vi "Read XML_Extra Checks_Check Parameter startBit Tx.vi"(8 "error in (no error)":errorcluster, 11 "Channels In":T1[](array[typedef])) -> (0 "error out":errorcluster)   [LabVIEW 2016]
doc: "This VI checks that for a given Hardware Channel, all parameters have a unique combination of Parameter settings: Hardware Channel, Label Decimal and Parameter Name. If there are multiple duplicates, the function returns all duplicates."
uses:
  XML_Channel.ctl
  XML_Label.ctl
  XML_Parameter.ctl
  <userlib>/_OpenG.lib/array/array.llb/Filter 1D Array with Scalar (Boolean)__ogtk.vi
panel:
  out "Error Source":string
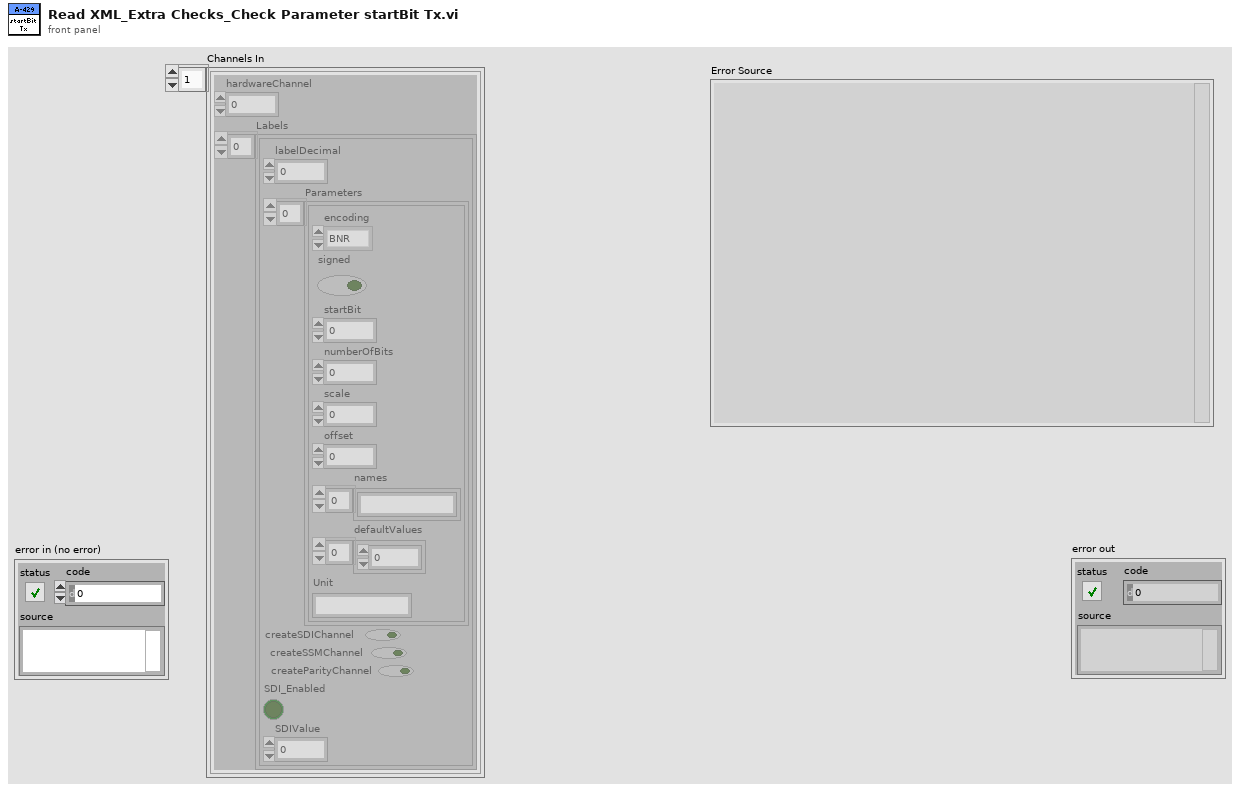
[diagram p1: front panel]
types:
  T1 = typedef "XML_Channel.ctl" = cluster{"hardwareChannel":i32, "Labels":T2[]}
  T2 = typedef "XML_Label.ctl" = cluster{"labelDecimal":i32, "Parameters":T3[], "createSDIChannel":bool, "createSSMChannel":bool, "createParityChannel":bool, "SDI_Enabled":bool, "SDIValue":u8}
  T3 = typedef "XML_Parameter.ctl" = cluster{"encoding":enum16{"BNR", "BCD", "Discrete"}, "signed":bool, "startBit":i32, "numberOfBits":i32, "scale":dbl, "offset":dbl, "names":string[], "defaultValues":dbl[], "Unit":string}
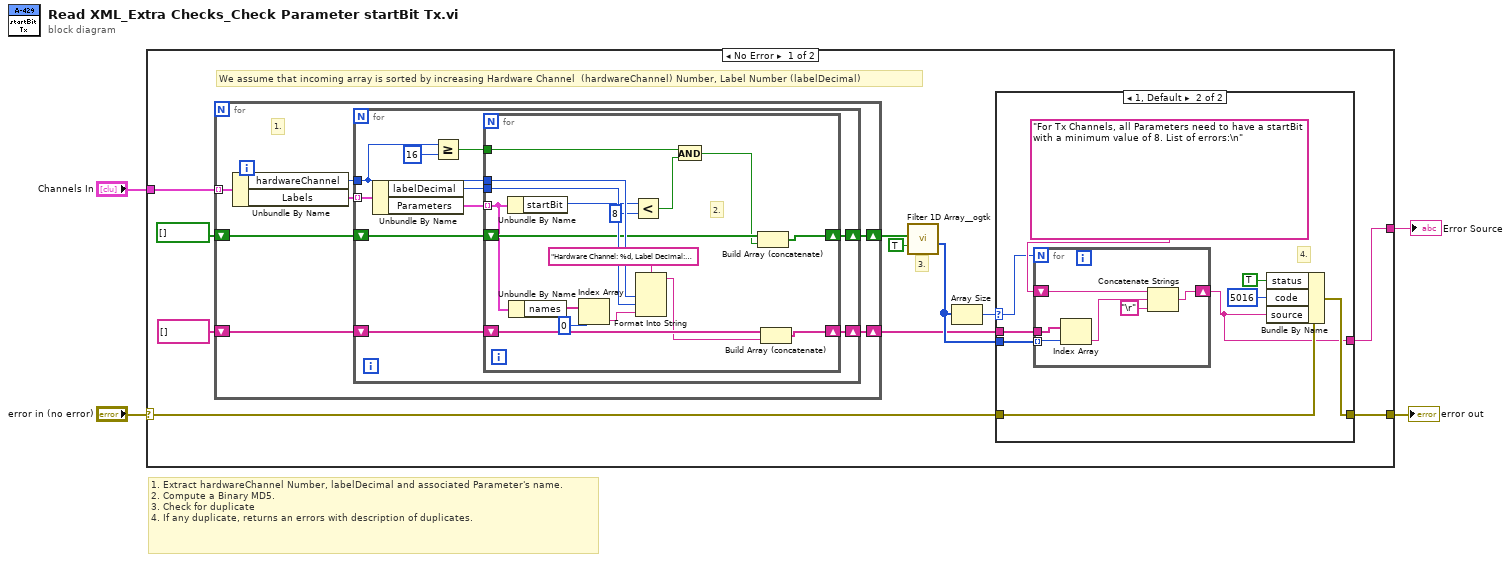
[diagram p0: block diagram]
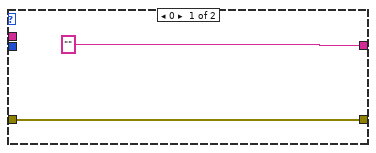
[diagram p2: hidden frame]
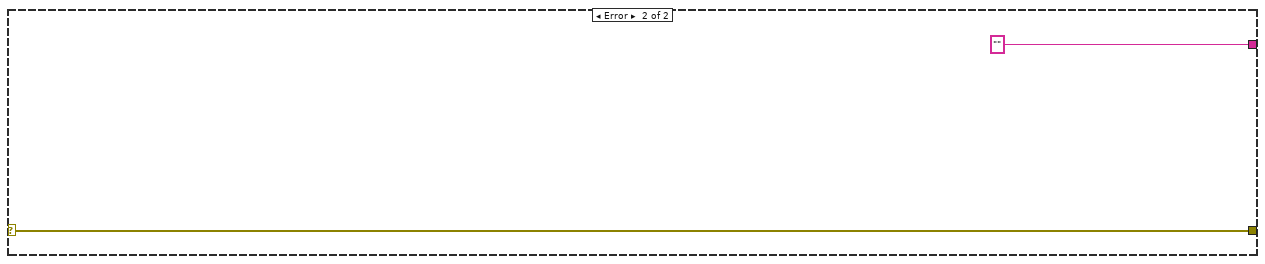
[diagram p3: hidden frame]
diagram:
  # "1. Extract hardwareChannel Number, labelDecimal and associated Parameter's name.\n2. Compute a Binary MD5.\n3. Check for duplicate\n4. If any duplicate, returns an errors with description of duplicates."
  n1 = case shown="No Error" "error in (no error)" {
    selector: "error in (no error)" -> [w14 w68]
    tunnel: [w11 w68] -> w3
    tunnel: "Channels In" -> [w13 _]
    tunnel: [w10 ""] -> w1
    frame No Error {
      # "3."
      # "We assume that incoming array is sorted by increasing Hardware Channel  (hardwareChannel) Number, Label Number (labelDecimal)"
      n2 = for {
        tunnel: w13 -> [w39] mode=indexing
        shift-right: [w35] -> w6
        shift-left: bool[] [] -> [w36]
        shift-right: [w33] -> w8
        shift-left: string[] [] -> [w34]
        # "1."
        n3 = Unbundle By Name(w39) -> ("hardwareChannel"=w38:i32, "Labels"=w37:T2[])
        n4 = for {
          tunnel: w38 -> [w42]
          tunnel: w37 -> [w49] mode=indexing
          shift-right: [w46] -> w35
          shift-left: w36 -> [w47]
          shift-right: [w43] -> w33
          shift-left: w34 -> [w44]
          n5 = Unbundle By Name(w49) -> ("labelDecimal"=w48:i32, "Parameters"=w45:T3[])
          n6 = Greater Or Equal?(x=w42, y=16) -> (x >= y?=w40:bool)
          n7 = for {
            tunnel: w42 -> [w66]
            tunnel: w48 -> [w65]
            shift-right: [w63] -> w46
            shift-left: w47 -> [w64]
            tunnel: w45 -> [w60] mode=indexing
            shift-right: [w61] -> w43
            shift-left: w44 -> [w62]
            tunnel: w40 -> [w54]
            # "2."
            n8 = Unbundle By Name(w60) -> ("startBit"=w53:i32)
            n9 = Unbundle By Name(w60) -> ("names"=w57:string[])
            n10 = Index Array(array=w57, index=0) -> (element=w56:string)
            n11 = Less?(x=w53, y=8) -> (x < y?=w51:bool)
            n12 = Format Into String(format string="Hardware Channel: %d, Label Decimal: %d, Name: %s", w66, w65, w56) -> (resulting string=w58:string)  [unwired: 2 in, 1 out]
            n13 = And(x=w54, y=w51) -> (x .and. y?=w50:bool)
            n14 = Build Array (concatenate)(w64, w50) -> (w63:bool[])
            n15 = Build Array (concatenate)(w62, w58) -> (w61:string[])
          }
        }
      }
      n16 = call-poly <userlib>:"Filter 1D Array__ogtk.vi"("items to filter"=TRUE, "array"=w6) -> ("filtered item indices"=w12:i32[])  [unwired: 4 in, 1 out]
      n17 = Array Size(array=w12) -> (size(s)=w15:i32)
      n18 = case shown="1, Default" w15 {
        selector: w15 -> [_ w21]
        tunnel: w14 -> [w17 w26]
        tunnel: w12 -> [_ w20]
        tunnel: [w17 w25] -> w11
        tunnel: ["" w19] -> w10
        tunnel: w8 -> [_ w18]
        frame 0 {
        }
        frame 1, Default {
          # "4."
          n19 = for {
            N: w21 -> [_]
            shift-right: [w31] -> w19
            shift-left: "For Tx Channels, all Parameters need to have a startBit with a minimum value of 8. List of errors:\n" -> [w32]
            tunnel: w20 -> [w30] mode=indexing
            tunnel: w18 -> [w28]
            n20 = Index Array(array=w28, index=w30) -> (element=w27:string)
            n21 = Concatenate Strings(w32, w27, "\r") -> (w31:string)
          }
          n22 = Bundle By Name(cluster=w26, "status"=TRUE, "code"=5016, "source"=w19) -> (w25:errorcluster)
        }
      }
    }
    frame Error {
    }
  }
  "error out" <- w3
  "Error Source" <- w1
